vi "Osc Query.vi"(0 "RedPitaya connection in":refnum<k5>, 2 "Query setting":u16(ring) items=["Voltage offset", "Voltage scale", "Probe attenuation", "Input gain", "Time offset", "Time scale", "Trigger sweep", "Trigger source", "Trigger slope", "Trigger level", "Data buffer size"], 5 "error in":errorcluster, 8 "Channel #":u16(ring) items=["Channel 1", "Channel 2"], 12 "timeout ms (2000)":i32) -> (14 "RedPitaya connection out":refnum<k5>, 16 "Output string":string, 19 "error out":errorcluster)   [LabVIEW 8.6]
doc: "Returns specific information from Red Pitaya. If the query is about parameters <b>vertical offset, vertical scale, probe attenuation, input gain</b>, you also have to provide the channel number."
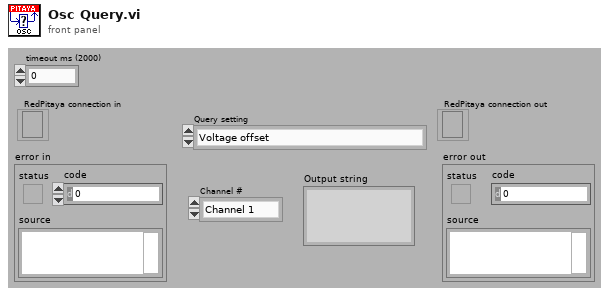
[diagram p1: front panel]
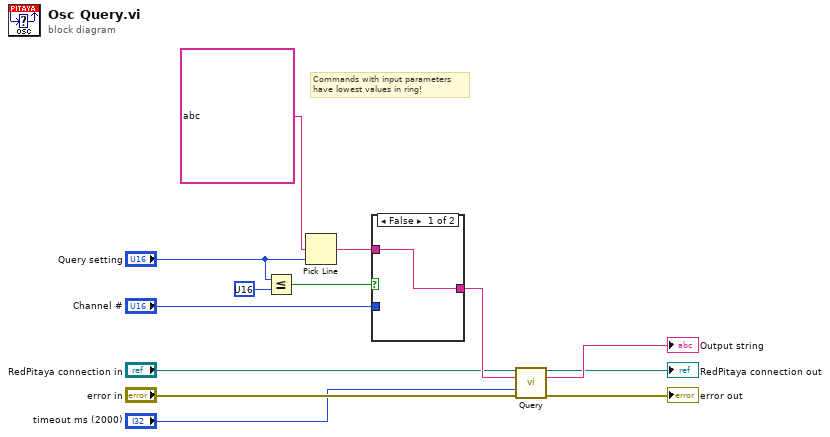
[diagram p0: block diagram]
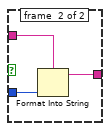
[diagram p2: hidden frame]
diagram:
  # "Commands with input parameters\nhave lowest values in ring!"
  n1 = Less Or Equal?(x="Query setting", y=u16 ?) -> (x <= y?=w10:bool)
  n2 = Pick Line(multi-line string=string ?, line index="Query setting") -> (output string=w7:string)  [unwired: 1 in]
  n3 = case shown="False" w10 {
    tunnel: [w14 w17] -> w11
    tunnel: "Channel #" -> [_ w16]
    tunnel: w7 -> [w14 w15]
    frame #0 {
    }
    frame #1 {
      n4 = Format Into String(format string=w15, w16) -> (resulting string=w17:string)  [unwired: 2 in, 1 out]
    }
  }
  n5 = call "Query.vi"("RedPitaya connection in"="RedPitaya connection in", "SCPI Query"=w11, "timeout ms (2000)"="timeout ms (2000)", "error in"="error in") -> ("RedPitaya connection out"=→"RedPitaya connection out":refnum<k5>, "data out"=→"Output string":string, "error out"=→"error out":errorcluster)  [unwired: 9 in]
